vi "CO calc loff.vi"(8 "CO conc":dbl, 9 "NO conc":dbl, 10 "NO:CO ratio":dbl, 11 "NOx MFR":dbl) -> (2 "CO MFR":dbl)   [LabVIEW 2014]
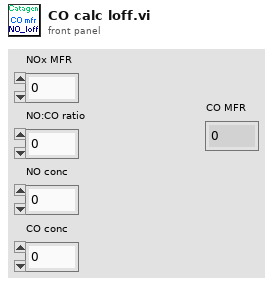
[diagram p1: front panel]
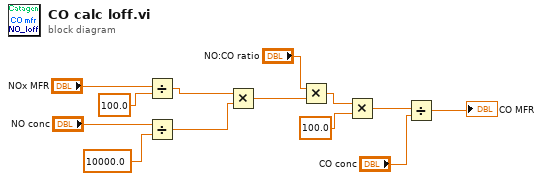
[diagram p0: block diagram]
diagram:
  n1 = Divide(x="NOx MFR", y=100.0) -> (x/y=w8:dbl)
  n2 = Divide(x="NO conc", y=10000.0) -> (x/y=w9:dbl)
  n3 = Multiply(x=w8, y=w9) -> (x*y=w6:dbl)
  n4 = Multiply(x="NO:CO ratio", y=w6) -> (x*y=w4:dbl)
  n5 = Multiply(x=w4, y=100.0 ("x*y")) -> (x*y=w3:dbl)
  n6 = Divide(x=w3, y="CO conc") -> (x/y=→"CO MFR":dbl)
